vi "ModifyNode.vi"(11 "Node":refnum<k20>) -> ()   [LabVIEW 2017]
uses:
  <vilib>/Utility/miscctls.llb/LVPoint32TypeDef.ctl
  <resource>/objmgr/DOMUserDefRef.rc
panel:
  out "Array":string[][](array[string])
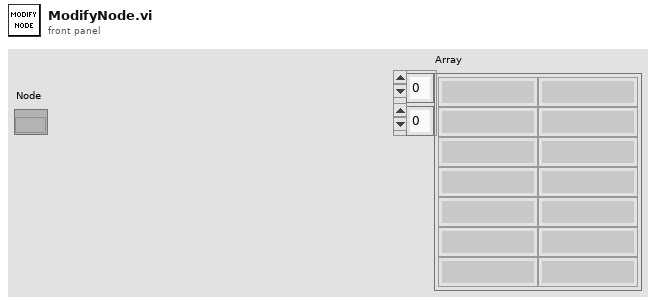
[diagram p1: front panel]
types:
  T1 = typedef "LVPoint32TypeDef.ctl" = cluster{"Horizontal":i32, "Vertical":i32}
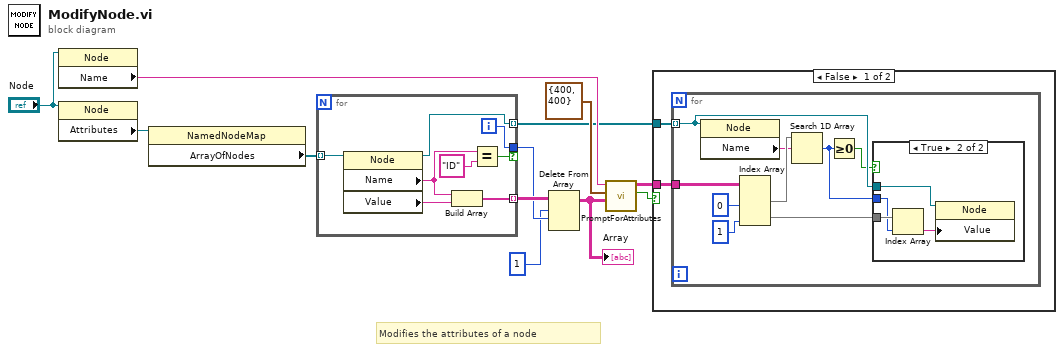
[diagram p0: block diagram]
diagram:
  # "Modifies the attributes of a node"
  n1 = property class="Node"(reference="Node") -> ("Name"=w6:string)  [unwired: 1 in, 2 out]
  n2 = property class="Node"(reference="Node") -> ("Attributes"=w12:refnum<k20>)  [unwired: 1 in, 2 out]
  n3 = property class="NamedNodeMap"(reference=w12) -> ("ArrayOfNodes"=w11:refnum<k20>[])  [unwired: 1 in, 2 out]
  n4 = for {
    tunnel: w11 -> [w16] mode=indexing
    tunnel: [w20] -> w10 mode=indexing
    tunnel: [w18] -> w9 if=w17
    tunnel: [w13] -> w3 mode=indexing
    i -> [w18]
    n5 = property class="Node"(reference=w16) -> (reference out=w13:refnum<k20>, "Name"=w15:string, "Value"=w14:string)  [unwired: 1 in, 1 out]
    n6 = Build Array(w15, w14) -> (w20:string[])
    n7 = Equal?(x=w15, y="ID") -> (x = y?=w17:bool)
  }
  n8 = Delete From Array(array=w10, length=1, index (row)=w9) -> (array with subset deleted=w5:string[][])  [unwired: 1 in, 1 out]
  "Array" <- w5
  n9 = call "PromptForAttributes.vi"("Attributes In"=w5, "Mouse Coords"=T1 {"Horizontal"=400, "Vertical"=400}, "New Node Name"=w6) -> ("Canceled"=w1:bool, "Attributes"=w2:string[][])  [unwired: 7 in]
  n10 = case shown="False" w1 {
    tunnel: w3 -> [w22 _]
    tunnel: w2 -> [w21 _]
    frame False {
      n11 = for {
        tunnel: w22 -> [w28] mode=indexing
        tunnel: w21 -> [w29]
        n12 = property class="Node"(reference=w28) -> ("Name"=w26:string)  [unwired: 1 in, 2 out]
        n13 = Index Array(array=w29, index (col) #1=0 ("disabled index (col)"), index (col) #2=1 ("index (col)")) -> (element #1=w27:string[], element #2=w25:string[])  [unwired: 2 in]
        n14 = Search 1D Array(1D array=w27, element=w26) -> (index of element=w24:i32)  [unwired: 1 in]
        n15 = Greater Or Equal To 0?(x=w24) -> (x >= 0?=w23:bool)
        n16 = case shown="True" w23 {
          tunnel: w28 -> [_ w35]
          tunnel: w25 -> [_ w34]
          tunnel: w24 -> [_ w32]
          frame False {
          }
          frame True {
            n17 = Index Array(array=w34, index=w32) -> (element=w33:string)
            n18 = property class="Node"(reference=w35, "Value"=w33) -> ()  [unwired: 1 in, 2 out]
          }
        }
      }
    }
    frame True {
    }
  }
